vi "uActor_Cleanup.vi"(8 "error in (no error)":errorcluster, 11 "uObserver in":refnum<class "uObserver.lvclass">) -> (0 "error out":errorcluster, 3 "uObserver out":refnum<class "uObserver.lvclass">)   [LabVIEW 2023, in "uFramework_pack_uActor.lvlib" / "uObserver.lvclass"]
doc: "The observer actor's cleanup routine retains the broker actor (which is owned by this observer) alive until all nested actors have affimatively stopped. This is to ensure other subscribers do not lose their observed broker before they have all shutdown gracefully."
uses:
  uObserver.lvclass
  uObserver.lvclass/uObserver.ctl
  Bin/uFramework.lvlibp/uActor/uActor.lvclass
  Bin/uFramework.lvlibp/uTransport_uActor/uTransport_uActor.lvclass
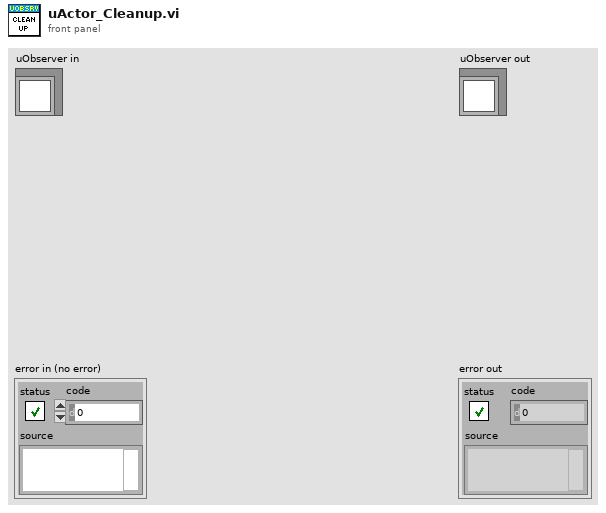
[diagram p1: front panel]
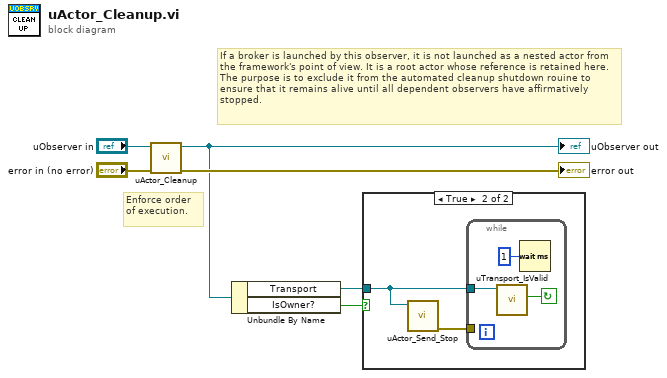
[diagram p0: block diagram]
diagram:
  # "Enforce order of execution."
  # "If a broker is launched by this observer, it is not launched as a nested actor from the framework's point of view. It is a root actor whose reference is retained here. The purpose is to exclude it from the automated cleanup shutdown rouine to ensure that it remains alive until all dependent observers have affirmatively stopped."
  n1 = call-parent "uActor_Cleanup.vi"("error in (no error)"="error in (no error)", "uActor in"="uObserver in") -> ("error out"=→"error out":errorcluster, "uActor out"=w3:refnum<class "uObserver.lvclass">)  [unwired: 8 in]
  "uObserver out" <- w3
  n2 = Unbundle By Name(w3) -> ("Transport"=w2:refnum<class "uTransport_uActor.lvclass">, "IsOwner?"=w1:bool)
  n3 = case shown="True" w1 {
    tunnel: w2 -> [_ w8]
    frame False {
    }
    frame True {
      n4 = call "uActor_Send_Stop.vi"("uActor Transport"=w8) -> ("error out"=w7:errorcluster)  [unwired: 10 in]
      n5 = while {
        tunnel: w8 -> [w11]
        tunnel: w7 -> [_]
        stop <- w10 continue-if-true
        n6 = call-dynamic "uTransport_IsValid.vi"("uTransport_uActor in"=w11) -> ("IsValid?"=w10:bool)  [unwired: 8 in, 2 out]
        n7 = Wait (ms)(milliseconds to wait=u32 1) -> ()  [unwired: 1 out]
      }
    }
  }
